vi "device registry.vi"(10 "device":u8, 11 "command":T1) -> (1 "Error?":bool, 2 "device out":u8)   [LabVIEW 2013, in "device.lvclass"]
uses:
  device.lvclass
  device registry command.ctl
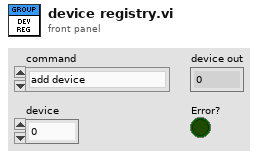
[diagram p1: front panel]
types:
  T1 = typedef "device.lvclass/device registry command.ctl" = enum16{"add device", "remove device", "get next available"}
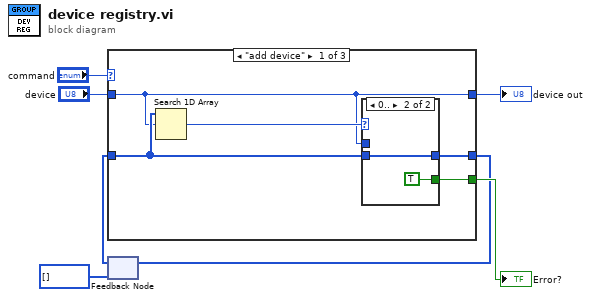
[diagram p0: block diagram]
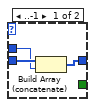
[diagram p2: hidden frame]
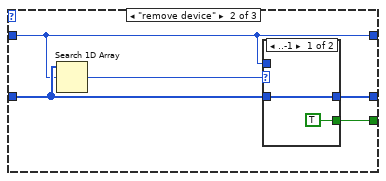
[diagram p3: hidden frame]
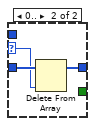
[diagram p4: hidden frame]
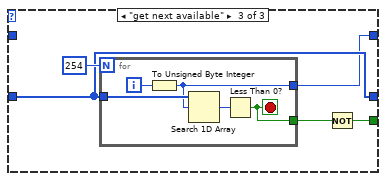
[diagram p5: hidden frame]
diagram:
  n1 = feedback #1(u8[] []) -> (w5:u8[])
  n2 = case shown="\"add device\"" "command" {
    tunnel: w5 -> [w10 w20 w31]
    tunnel: "device" -> [w8 w18 _]
    tunnel: [w11 w21 w28] -> w3
    tunnel: [w9 w19 w31] -> w2
    tunnel: [w8 w18 w30] -> w1
    frame "add device" {
      n3 = Search 1D Array(1D array=w10, element=w8) -> (index of element=w12:i32)  [unwired: 1 in]
      n4 = case shown="0.." w12 {
        tunnel: [_ TRUE] -> w11
        tunnel: w10 -> [w15 w16]
        tunnel: w8 -> [w14 _]
        tunnel: [w13 w16] -> w9
        frame ..-1 {
          n5 = Build Array (concatenate)(w15, w14) -> (w13:u8[])
        }
        frame 0.. {
        }
      }
    }
    frame "remove device" {
      n6 = Search 1D Array(1D array=w20, element=w18) -> (index of element=w22:i32)  [unwired: 1 in]
      n7 = case shown="..-1" w22 {
        selector: w22 -> [_ w26]
        tunnel: [TRUE _] -> w21
        tunnel: w20 -> [w23 w27]
        tunnel: w18 -> [_ _]
        tunnel: [w23 w25] -> w19
        frame ..-1 {
        }
        frame 0.. {
          n8 = Delete From Array(array=w27, index=w26) -> (array with subset deleted=w25:u8[])  [unwired: 1 in, 1 out]
        }
      }
    }
    frame "get next available" {
      n9 = for {
        N: 254 -> [_]
        tunnel: w31 -> [w36]
        tunnel: [w34] -> w30
        tunnel: [w33] -> w29
        i -> [w37]
        stop <- w33 stop-if-true
        n10 = To Unsigned Byte Integer(number=w37) -> (unsigned 8bit integer=w34:u8)
        n11 = Search 1D Array(1D array=w36, element=w34) -> (index of element=w35:i32)  [unwired: 1 in]
        n12 = Less Than 0?(x=w35) -> (x < 0?=w33:bool)
      }
      n13 = Not(x=w29) -> (.not. x?=w28:bool)
    }
  }
  "Error?" <- w3
  "device out" <- w1
  n14 = feedback-in #1(w2) -> ()
